vi "get sender.vi"(11 "message in":refnum<class "communicator message.lvclass">) -> (2 "invalid?":bool, 3 "sender":refnum<class "identifying queue.lvclass">)   [LabVIEW 2015, in "communicator message.lvclass"]
uses:
  communicator message.lvclass
  communicator queue/identifying queue.lvclass
  communicator message.lvclass/communicator message.ctl
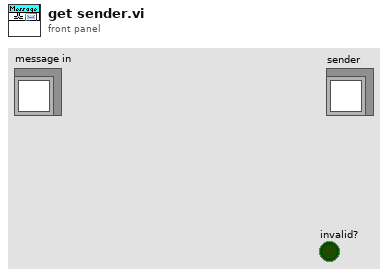
[diagram p1: front panel]
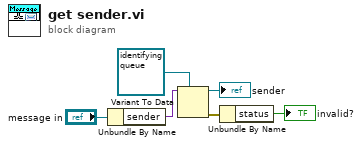
[diagram p0: block diagram]
diagram:
  n1 = Unbundle By Name("message in") -> ("sender"=w5:variant)
  n2 = Variant To Data(type=refnum<class "identifying queue.lvclass"> refnum ("sender 2"), Variant=w5) -> (data=→"sender":refnum<class "identifying queue.lvclass">, error out=w2:errorcluster)  [unwired: 1 in]
  n3 = Unbundle By Name(w2) -> ("status"=→"invalid?":bool)
